vi "DFD Save to File.vi"   [LabVIEW 2017, in "NI_DigFilterLicensed.lvlib"]
doc: "Saves a filter or a filter bank into a file. Wire data to the <B>filter in</B> input to determine the polymorphic instance to use or manually select the instance."
uses:
  <vilib>/addons/Digital Filter Design/NI_DigFilterLicensed.lvlib
  <vilib>/addons/Digital Filter Design/NI_DigFilter_FilterBank.lvlib
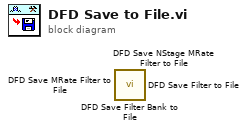
[diagram p0: block diagram]
diagram:
  n1 = call <vilib>:"DFD Save Filter Bank to File.vi"() -> ()  [unwired: 9 in, 3 out]
  n2 = call <vilib>:"DFD Save NStage MRate Filter to File.vi"() -> ()  [unwired: 9 in, 3 out]
  n3 = call <vilib>:"DFD Save MRate Filter to File.vi"() -> ()  [unwired: 9 in, 3 out]
  n4 = call <vilib>:"DFD Save Filter to File.vi"() -> ()  [unwired: 9 in, 3 out]
